vi "FM_RTL-SDR_RX-DLL_X32.vi"() -> ()   [LabVIEW 2013]
uses:
  <vilib>/sound2/lvsound2.llb/Sound Data Format.ctl
  <vilib>/Analysis/2dsp.llb/Decimate (single shot, DBL).vi
  <vilib>/sound2/lvsound2.llb/Sound Output Write (DBL Single).vi
  <vilib>/Analysis/NI_AALPro.lvlib
panel:
  in  "SampleFrequencyMHz":dbl=2.0 format="%#_13g"
  in  "reference":refnum<k24>
  in  "Device index":i32
  in  "CarrierFrequencyMHz":dbl=104.3
  out "Boolean":bool
  out "error out":errorcluster
  out "error out":errorcluster
  out "error out":errorcluster
  in  "sound format":T1={"sample rate (S/s)"=44100.0, "number of channels"=1, "bits per sample"=16}
  in  "stop":bool
  out "error out":errorcluster
  # "FM Receiver"
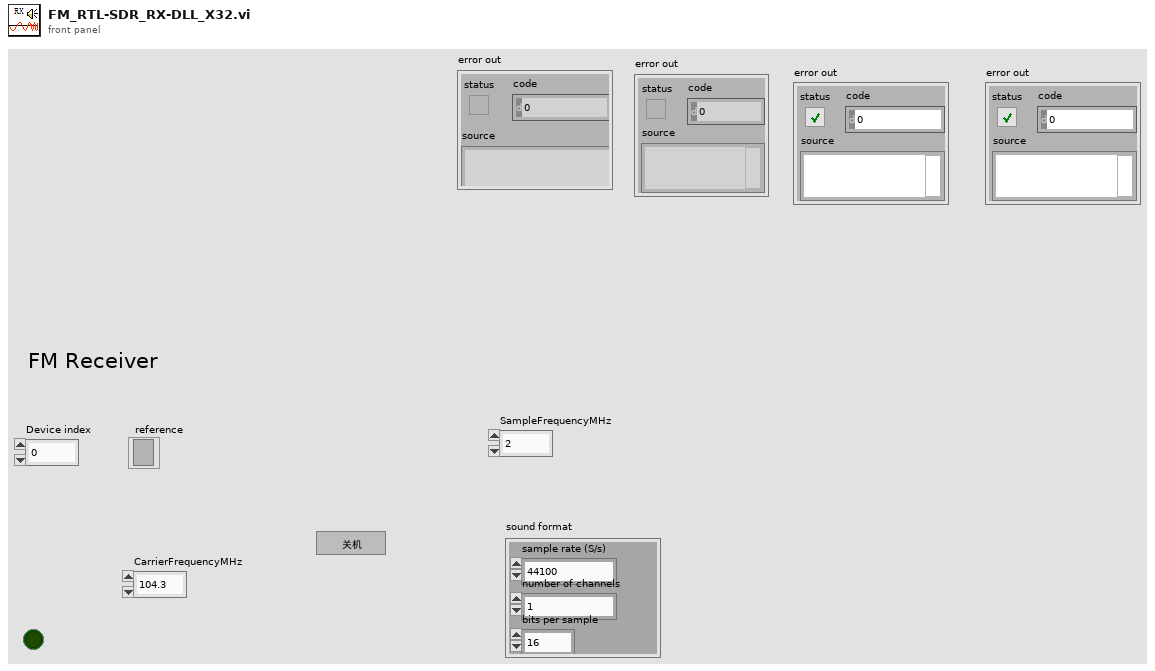
[diagram p1: front panel]
types:
  T1 = typedef "Sound Data Format.ctl" = cluster{"sample rate (S/s)":dbl, "number of channels":i32, "bits per sample":i32}
  T2 = typedef "Sound Output Task ID.ctl" = u32
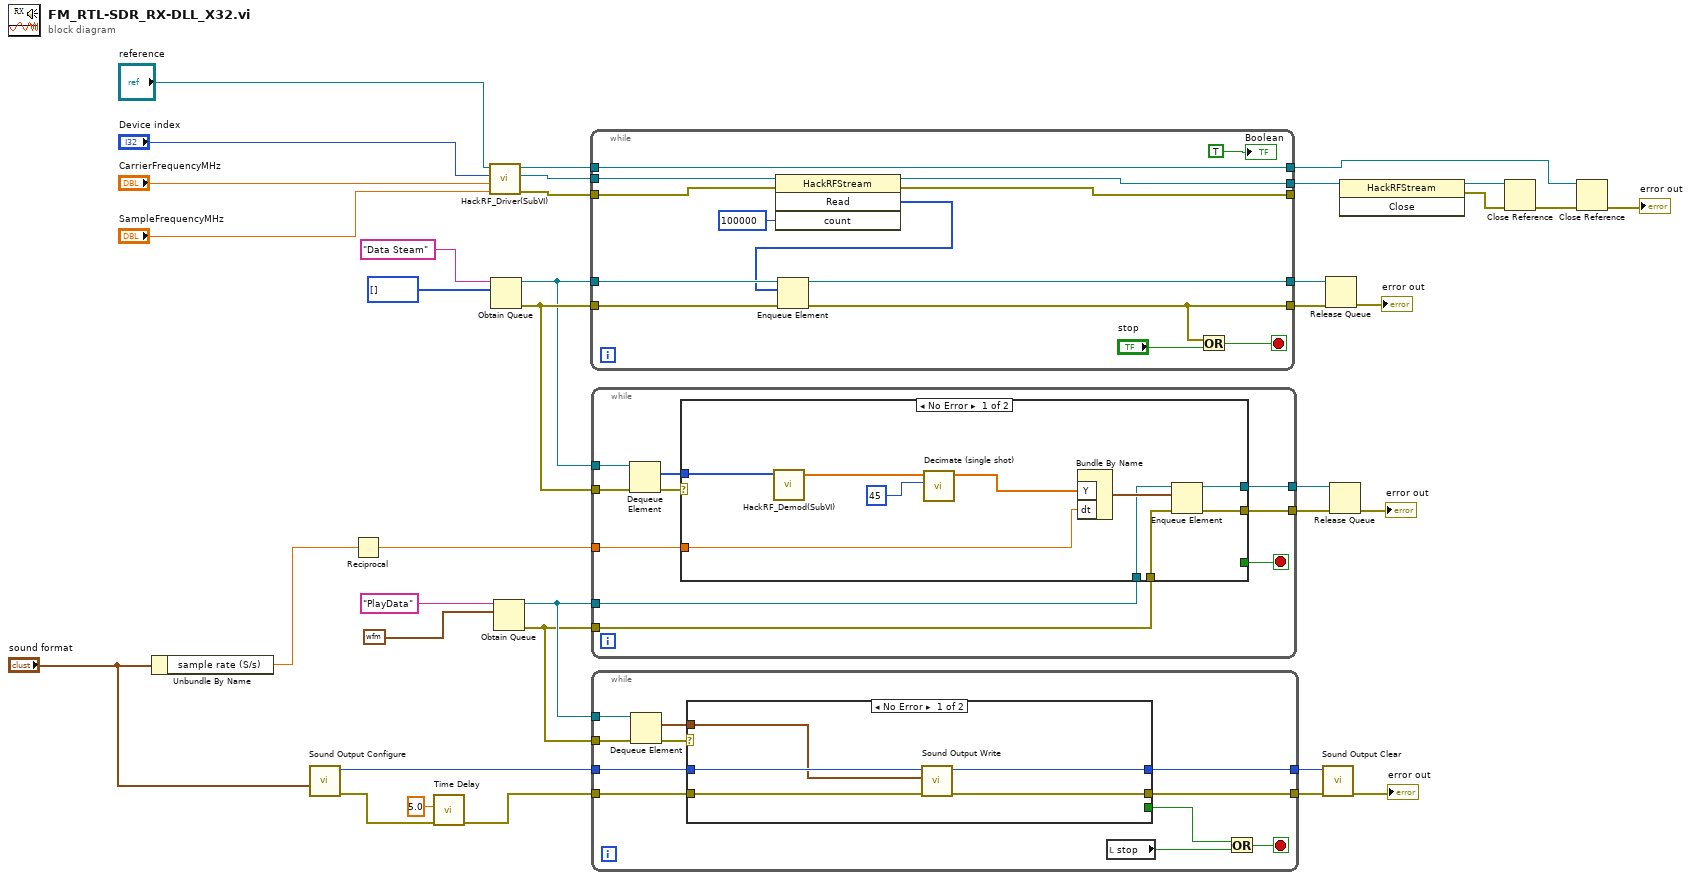
[diagram p0: block diagram]
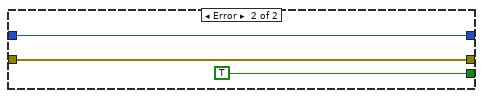
[diagram p2: hidden frame]
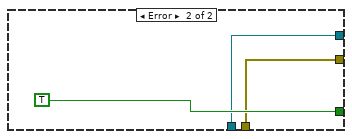
[diagram p3: hidden frame]
diagram:
  n1 = Unbundle By Name("sound format") -> ("sample rate (S/s)"=w2:dbl)
  n2 = call <vilib>:"Sound Output Configure.vi"("sound format"="sound format") -> ("error out"=w31:errorcluster, "task ID"=w25:T2)  [unwired: 9 in]
  n3 = Reciprocal(x=w2) -> (1/x=w1:dbl)
  n4 = call "Time Delay"("error in (no error)"=w31, "Delay Time (s)"=5.0) -> ("error out"=w22:errorcluster)  [unwired: 9 in]
  n5 = call "HackRF_Driver(SubVI).vi"("SampleFrequencyMHz"="SampleFrequencyMHz", "CarrierFrequencyMHz"="CarrierFrequencyMHz", "Device index"="Device index", ".NET Refnum in"="reference") -> ("error out"=w11:errorcluster, "StartRX"=w10:refnum<k24>, ".NET Refnum out"=w12:refnum<k24>)  [unwired: 5 in]
  n6 = Obtain Queue(name (unnamed)="Data Steam", element data type=u8[] [] ("buf 2")) -> (queue out=w28:refnum<queue>, error out=w29:errorcluster)  [unwired: 3 in, 1 out]
  n7 = Obtain Queue(name (unnamed)="PlayData", element data type=waveform(dbl) {"t0"=timestamp(0 s since 1904-01-01), "dt"=1.0, "Y"=[]} ("waveform")) -> (queue out=w23:refnum<queue>, error out=w19:errorcluster)  [unwired: 3 in, 1 out]
  n8 = while {
    tunnel: w28 -> [w51]
    tunnel: [w50] -> w34
    tunnel: w29 -> [w49]
    tunnel: [w48] -> w33
    tunnel: w12 -> [w40]
    tunnel: w11 -> [w43]
    tunnel: [w42] -> _
    tunnel: w10 -> [w41]
    tunnel: [w40] -> w5
    tunnel: [w39] -> w4
    stop <- w46 stop-if-true
    n9 = invoke class="HackRFStream" method="Read"(reference=w41, error in=w43, "count"=100000) -> (reference out=w39:refnum<k24>, error out=w42:errorcluster, "Read"=w44:u8[])  [unwired: 1 in, 1 out]
    n10 = Enqueue Element(queue=w51, element=w44, error in (no error)=w49) -> (queue out=w50:refnum<queue>, error out=w48:errorcluster)  [unwired: 1 in, 1 out]
    n11 = Or(x=w48, y="stop") -> (x .or. y?=w46:bool)
    "Boolean" <- TRUE
  }
  n12 = while {
    tunnel: w28 -> [w61]
    tunnel: w29 -> [w59]
    tunnel: w23 -> [w56]
    tunnel: w19 -> [w55]
    tunnel: [w54] -> w17
    tunnel: [w53] -> w16
    tunnel: w1 -> [w52]
    stop <- w57 stop-if-true
    n13 = Dequeue Element(queue=w61, error in (no error)=w59) -> (element=w60:u8[], error out=w58:errorcluster)  [unwired: 1 in, 2 out]
    n14 = case shown="No Error" w58 {
      tunnel: w60 -> [w66 _]
      tunnel: [_ TRUE] -> w57
      tunnel: w56 -> [w70 w73]
      tunnel: w55 -> [w69 w72]
      tunnel: [w68 w73] -> w54
      tunnel: [w67 w72] -> w53
      tunnel: w52 -> [w62 _]
      frame No Error {
        n15 = call "HackRF_Demod(SubVI).vi"("Read"=w66) -> ("dX/dt"=w64:dbl[])  [unwired: 10 in]
        n16 = call-poly <vilib>:"Decimate (single shot).vi"("decimating factor"=45, "X"=w64) -> ("Decimated Array"=w63:dbl[])  [unwired: 8 in, 1 out]
        n17 = Bundle By Name ("Build Waveform")("Y"=w63, "dt"=w62) -> (w71:waveform(dbl))  [unwired: 1 in]
        n18 = Enqueue Element(queue=w70, element=w71, error in (no error)=w69) -> (queue out=w68:refnum<queue>, error out=w67:errorcluster)  [unwired: 1 in, 1 out]
      }
      frame Error {
      }
    }
  }
  n19 = while {
    tunnel: w25 -> [w85]
    tunnel: [w84] -> w24
    tunnel: w23 -> [w83]
    tunnel: w19 -> [w82]
    tunnel: w22 -> [w81]
    tunnel: [w80] -> w21
    stop <- w75 stop-if-true
    n20 = Dequeue Element(queue=w83, error in (no error)=w82) -> (element=w78:waveform(dbl), error out=w79:errorcluster)  [unwired: 1 in, 2 out]
    n21 = case shown="No Error" w79 {
      tunnel: w85 -> [w90 w93]
      tunnel: [w89 w93] -> w84
      tunnel: w81 -> [w88 w92]
      tunnel: [w87 w92] -> w80
      tunnel: w78 -> [w86 _]
      tunnel: [_ TRUE] -> w77
      frame No Error {
        n22 = call-poly <vilib>:"Sound Output Write.vi"("error in (no error)"=w88, "data"=w86, "task ID"=w90) -> ("error out"=w87:errorcluster, "task ID out"=w89:T2)  [unwired: 7 in]
      }
      frame Error {
      }
    }
    n23 = local read "stop"() -> (w76:bool)
    n24 = Or(x=w77, y=w76) -> (x .or. y?=w75:bool)
  }
  n25 = call <vilib>:"Sound Output Clear.vi"("error in (no error)"=w21, "task ID"=w24) -> ("error out"=→"error out":errorcluster)  [unwired: 9 in]
  n26 = Release Queue(queue=w34, error in (no error)=w33) -> (error out=→"error out":errorcluster)  [unwired: 1 in, 2 out]
  n27 = Release Queue(queue=w17, error in (no error)=w16) -> (error out=→"error out":errorcluster)  [unwired: 1 in, 2 out]
  n28 = invoke class="HackRFStream" method="Close"(reference=w4) -> (reference out=w9:refnum<k24>, error out=w8:errorcluster)  [unwired: 2 in, 1 out]
  n29 = Close Reference(reference=w9, error in (no error)=w8) -> (error out=w7:errorcluster)
  n30 = Close Reference(reference=w5, error in (no error)=w7) -> (error out=→"error out":errorcluster)
